vi "createTelemetryFPGAData.vi"(8 "error in (no error)":errorcluster, 11 "UserEvents in":refnum<class "UserEvents.lvclass">) -> (0 "error out":errorcluster, 3 "UserEvents out":refnum<class "UserEvents.lvclass">)   [LabVIEW 2016, in "UserEvents.lvclass"]
uses:
  UserEvents.lvclass
  DataTypes/Topics/TelemetryFPGAData.ctl
  DataTypes/Topics/Parts/Timestamp.ctl
  UserEvents.lvclass/UserEvents.ctl
  DataTypes/Topics/M1M3SupportTopics.lvlib
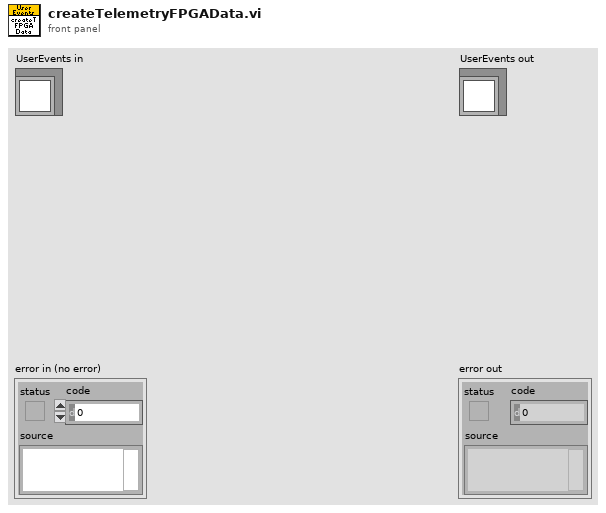
[diagram p1: front panel]
types:
  T1 = typedef "M1M3SupportTopics.lvlib/TelemetryFPGAData.ctl" = cluster{"Timestamp":T2, "ModbusSubnetATxInternalFIFOOverflow":bool, "ModbusSubnetAInvalidInstruction":bool, "ModbusSubnetAWaitForRxFrameTimeout":bool, "ModbusSubnetAStartBitError":bool, "ModbusSubnetAStopBitError":bool, "ModbusSubnetARxDataFIFOOverflow":bool, "ModbusSubnetATxByteCount":u32, "ModbusSubnetATxFrameCount":u32, "ModbusSubnetARxByteCount":u32, "ModbusSubnetARxFrameCount":u32, "ModbusSubnetBTxInternalFIFOOverflow":bool, "ModbusSubnetBInvalidInstruction":bool, "ModbusSubnetBWaitForRxFrameTimeout":bool, "ModbusSubnetBStartBitError":bool, "ModbusSubnetBStopBitError":bool, "ModbusSubnetBRxDataFIFOOverflow":bool, "ModbusSubnetBTxByteCount":u32, "ModbusSubnetBTxFrameCount":u32, "ModbusSubnetBRxByteCount":u32, "ModbusSubnetBRxFrameCount":u32, "ModbusSubnetCTxInternalFIFOOverflow":bool, "ModbusSubnetCInvalidInstruction":bool, "ModbusSubnetCWaitForRxFrameTimeout":bool, "ModbusSubnetCStartBitError":bool, "ModbusSubnetCStopBitError":bool, "ModbusSubnetCRxDataFIFOOverflow":bool, "ModbusSubnetCTxByteCount":u32, "ModbusSubnetCTxFrameCount":u32, "ModbusSubnetCRxByteCount":u32, "ModbusSubnetCRxFrameCount":u32, "ModbusSubnetDTxInternalFIFOOverflow":bool, "ModbusSubnetDInvalidInstruction":bool, "ModbusSubnetDWaitForRxFrameTimeout":bool, "ModbusSubnetDStartBitError":bool, "ModbusSubnetDStopBitError":bool, "ModbusSubnetDRxDataFIFOOverflow":bool, "ModbusSubnetDTxByteCount":u32, "ModbusSubnetDTxFrameCount":u32, "ModbusSubnetDRxByteCount":u32, "ModbusSubnetDRxFrameCount":u32, "ModbusSubnetETxInternalFIFOOverflow":bool, "ModbusSubnetEInvalidInstruction":bool, "ModbusSubnetEWaitForRxFrameTimeout":bool, "ModbusSubnetEStartBitError":bool, "ModbusSubnetEStopBitError":bool, "ModbusSubnetERxDataFIFOOverflow":bool, "ModbusSubnetETxByteCount":u32, "ModbusSubnetETxFrameCount":u32, "ModbusSubnetERxByteCount":u32, "ModbusSubnetERxFrameCount":u32, "FPGATimestamp":dbl}
  T2 = typedef "M1M3SupportTopics.lvlib/Timestamp.ctl" = dbl
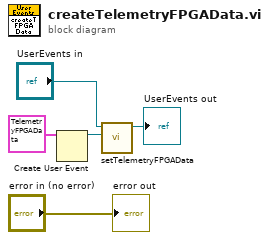
[diagram p0: block diagram]
diagram:
  n1 = Create User Event(user event datatype=T1 {"Timestamp"=0.0, "ModbusSubnetATxInternalFIFOOverflow"=FALSE, "ModbusSubnetAInvalidInstruction"=FALSE, "ModbusSubnetAWaitForRxFrameTimeout"=FALSE, "ModbusSubnetAStartBitError"=FALSE, "ModbusSubnetAStopBitError"=FALSE, "ModbusSubnetARxDataFIFOOverflow"=FALSE, "ModbusSubnetATxByteCount"=0, "ModbusSubnetATxFrameCount"=0, "ModbusSubnetARxByteCount"=0, "ModbusSubnetARxFrameCount"=0, "ModbusSubnetBTxInternalFIFOOverflow"=FALSE, "ModbusSubnetBInvalidInstruction"=FALSE, "ModbusSubnetBWaitForRxFrameTimeout"=FALSE, "ModbusSubnetBStartBitError"=FALSE, "ModbusSubnetBStopBitError"=FALSE, "ModbusSubnetBRxDataFIFOOverflow"=FALSE, "ModbusSubnetBTxByteCount"=0, "ModbusSubnetBTxFrameCount"=0, "ModbusSubnetBRxByteCount"=0, "ModbusSubnetBRxFrameCount"=0, "ModbusSubnetCTxInternalFIFOOverflow"=FALSE, "ModbusSubnetCInvalidInstruction"=FALSE, "ModbusSubnetCWaitForRxFrameTimeout"=FALSE, "ModbusSubnetCStartBitError"=FALSE, "ModbusSubnetCStopBitError"=FALSE, "ModbusSubnetCRxDataFIFOOverflow"=FALSE, "ModbusSubnetCTxByteCount"=0, "ModbusSubnetCTxFrameCount"=0, "ModbusSubnetCRxByteCount"=0, "ModbusSubnetCRxFrameCount"=0, "ModbusSubnetDTxInternalFIFOOverflow"=FALSE, "ModbusSubnetDInvalidInstruction"=FALSE, "ModbusSubnetDWaitForRxFrameTimeout"=FALSE, "ModbusSubnetDStartBitError"=FALSE, "ModbusSubnetDStopBitError"=FALSE, "ModbusSubnetDRxDataFIFOOverflow"=FALSE, "ModbusSubnetDTxByteCount"=0, "ModbusSubnetDTxFrameCount"=0, "ModbusSubnetDRxByteCount"=0, "ModbusSubnetDRxFrameCount"=0, "ModbusSubnetETxInternalFIFOOverflow"=FALSE, "ModbusSubnetEInvalidInstruction"=FALSE, "ModbusSubnetEWaitForRxFrameTimeout"=FALSE, "ModbusSubnetEStartBitError"=FALSE, "ModbusSubnetEStopBitError"=FALSE, "ModbusSubnetERxDataFIFOOverflow"=FALSE, "ModbusSubnetETxByteCount"=0, "ModbusSubnetETxFrameCount"=0, "ModbusSubnetERxByteCount"=0, "ModbusSubnetERxFrameCount"=0, "FPGATimestamp"=0.0} ("TelemetryFPGAData")) -> (user event=w2:refnum<user-event>)  [unwired: 1 in, 1 out]
  n2 = call "setTelemetryFPGAData.vi"("TelemetryFPGAData"=w2, "UserEvents in"="UserEvents in") -> ("UserEvents out"=→"UserEvents out":refnum<class "UserEvents.lvclass">)  [unwired: 9 in]
  "error out" <- "error in (no error)"
